vi "Auto 10.vi"(8 "Error In":errorcluster) -> (0 "Error Out":errorcluster)   [LabVIEW 2014]
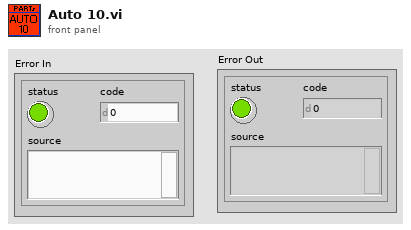
[diagram p1: front panel]
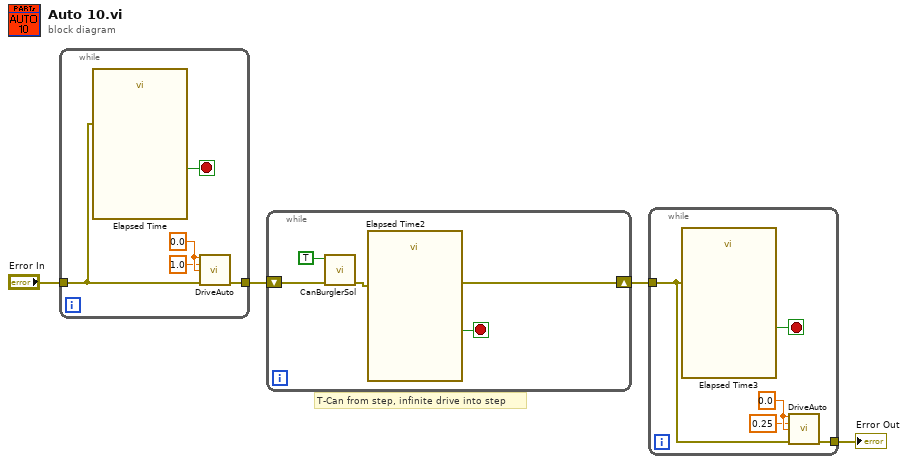
[diagram p0: block diagram]
diagram:
  # "T-Can from step, infinite drive into step"
  n1 = while {
    tunnel: [w9] -> w4
    tunnel: "Error In" -> [w6]
    stop <- w7 stop-if-true
    w8 = 0.0 ("Arm Value")
    n2 = call "Elapsed Time"("error in (no error)"=w6) -> ("Time has Elapsed"=w7:bool)  [unwired: 11 in, 7 out]
    n3 = call "DriveAuto.vi"("X In"=w8, "Y In"=1.0 ("X In"), "R In"=w8, "Error In"=w6) -> ("Error Out"=w9:errorcluster)  [unwired: 11 in]
  }
  n4 = while {
    shift-right: [w12] -> w3
    shift-left: w4 -> [w14]
    stop <- w11 stop-if-true
    n5 = call "CanBurglerSol.vi"("Error In"=w14, "Grabber Open/Close"=TRUE) -> ("Error Out"=w13:errorcluster)  [unwired: 9 in]
    n6 = call "Elapsed Time2"("error in (no error)"=w13) -> ("Time has Elapsed"=w11:bool, "error out"=w12:errorcluster)  [unwired: 11 in, 6 out]
  }
  n7 = while {
    tunnel: [w19] -> w1
    tunnel: w3 -> [w16]
    stop <- w17 stop-if-true
    w18 = 0.0 ("Arm Value")
    n8 = call "Elapsed Time3"("error in (no error)"=w16) -> ("Time has Elapsed"=w17:bool)  [unwired: 11 in, 7 out]
    n9 = call "DriveAuto.vi"("X In"=w18, "Y In"=0.25 ("X In"), "R In"=w18, "Error In"=w16) -> ("Error Out"=w19:errorcluster)  [unwired: 11 in]
  }
  "Error Out" <- w1
